vi "G#Object_GetClassVersion.vi"(0 "reference in":refnum<class "G#Object.lvclass">, 5 "error in (no error)":errorcluster) -> (14 "reference out":refnum<class "G#Object.lvclass">, 16 "version":string, 19 "error out":errorcluster)   [LabVIEW 2017, in "G#Object.lvclass"]
doc: "Returns the version of the class specified by reference in."
uses:
  G#Object.lvclass
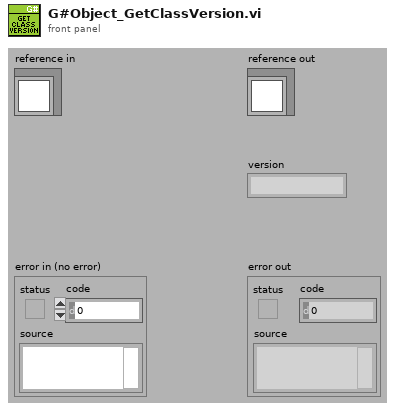
[diagram p1: front panel]
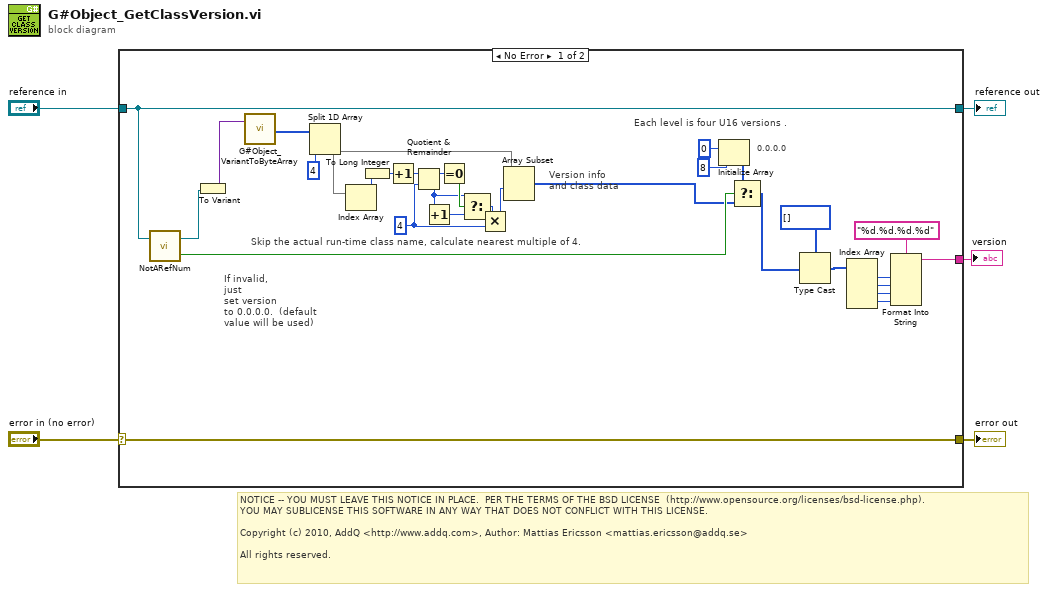
[diagram p0: block diagram]
diagram:
  # "NOTICE -- YOU MUST LEAVE THIS NOTICE IN PLACE.  PER THE TERMS OF THE BSD LICENSE  (http://www.opensource.org/licenses/bsd-license.php).\nYOU MAY SUBLICENSE THIS SOFTWARE IN ANY WAY THAT DOES NOT CONFLICT WITH THIS LICENSE.\n\nCopyright (c) 2010, AddQ <http://www.addq.com>, Author: Mattias Ericsson <mattias.ericsson@addq.se>\n\nAll rights reserved."
  n1 = case shown="No Error" "error in (no error)" {
    selector: "error in (no error)" -> [w19 w38]
    tunnel: [w19 w38] -> w4
    tunnel: [w21 w37] -> w2
    tunnel: "reference in" -> [w21 w37]
    tunnel: [w8 _] -> w1
    frame No Error {
      w28 = 4 ("y")
      # "0.0.0.0"
      # "If invalid,\njust\nset version\nto 0.0.0.0.  (default\nvalue will be used)"
      # "Each level is four U16 versions ."
      # "Version info\nand class data"
      # "Skip the actual run-time class name, calculate nearest multiple of 4."
      n2 = call-dynamic "NotARefNum.vi"("reference in"=w21) -> ("not a refnum?"=w20:bool, "reference out"=w22:refnum<class "G#Object.lvclass">)  [unwired: 1 in]
      n3 = To Variant(anything=w22) -> (Variant=w7:variant)
      n4 = call "G#Object_VariantToByteArray.vi"("variant"=w7) -> ("unsigned byte array"=w6:u8[])  [unwired: 17 in, 1 out]
      n5 = Split 1D Array(array=w6, index=4 ("length")) -> (second subarray=w27:u8[])  [unwired: 1 out]
      n6 = Index Array(array=w27) -> (element=w36:u8)  [unwired: 1 in]
      n7 = To Long Integer(number=w36) -> (32bit integer=w26:i32)
      n8 = Increment(x=w26) -> (x+1=w25:i32)
      n9 = Quotient & Remainder(x=w25, y=w28) -> (x-y*floor(x/y)=w35:i32, floor(x/y)=w32:i32)
      n10 = Increment(x=w32) -> (x+1=w33:i32)
      n11 = Equal To 0?(x=w35) -> (x = 0?=w34:bool)
      n12 = Select(t=w32, s=w34, f=w33) -> (s? t:f=w30:i32)
      n13 = Multiply(x=w30, y=w28) -> (x*y=w29:i32)
      n14 = Array Subset(array=w27, index=w29) -> (w18:u8[])  [unwired: 1 in]
      n15 = Initialize Array(u8 0, 8 ("dimension size")) -> (w24:u8[])
      n16 = Select(t=w24, s=w20, f=w18) -> (s? t:f=w16:u8[])
      n17 = Type Cast(type=u16[] [], x=w16) -> (*(type *) &x=w14:u16[])
      n18 = Index Array(array=w14) -> (element #1=w13:u16, element #2=w12:u16, element #3=w11:u16, element #4=w10:u16)  [unwired: 4 in]
      n19 = Format Into String(format string="%d.%d.%d.%d", w13, w12, w11, w10) -> (resulting string=w8:string)  [unwired: 2 in, 1 out]
    }
    frame Error {
    }
  }
  "error out" <- w4
  "reference out" <- w2
  "version" <- w1
